vi "子VI-数据库显示.vi"(10 "数据库保存路径":path, 11 "表名":string) -> (2 "Table":string[][](table) caption="表格")   [LabVIEW 2018]
uses:
  <vilib>/addons/database/_DB Variant To Data/Database Variant To Data.xnode
  <vilib>/addons/database/Connection.llb/DB Tools Open Connec (String).vi
  <vilib>/addons/database/NI_Database_API.lvlib
panel:
  out "data":string[][](array[string])
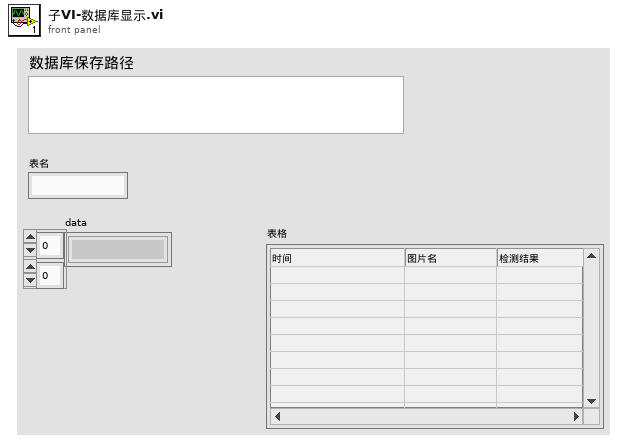
[diagram p1: front panel]
types:
  T1 = typedef "NI_Database_API.lvlib/Conn ObjectReference.ctl" = refnum<k1>
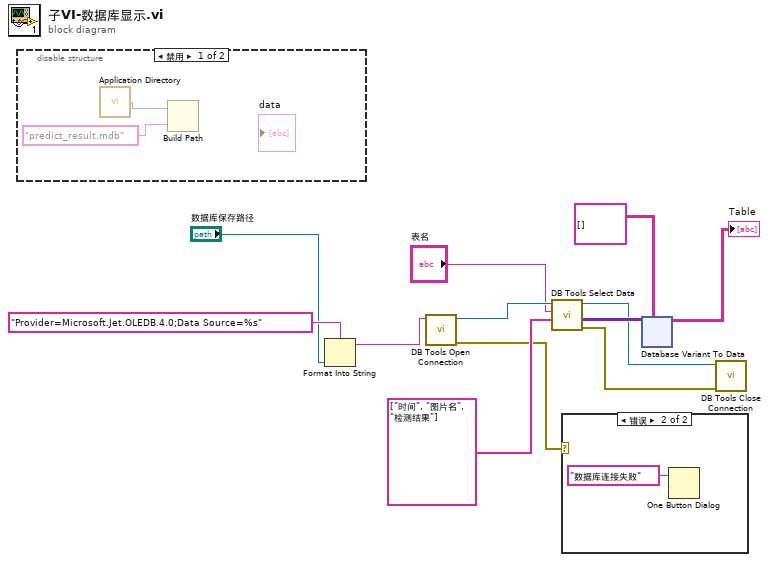
[diagram p0: block diagram]
diagram:
  n1 = disable-structure shown="禁用" {
    frame Disabled {
      n2 = call <vilib>:"Application Directory.vi"() -> ("Application Directory"=w14:path)
      n3 = Build Path(base path=w14, name or relative path="predict_result.mdb" ("名称或相对路径")) -> ()  [unwired: 1 out]
    }
    frame Enabled {
    }
  }
  n4 = Format Into String(format string="Provider=Microsoft.Jet.OLEDB.4.0;Data Source=%s" ("格式字符串"), "数据库保存路径") -> (resulting string=w4:string)  [unwired: 2 in, 1 out]
  n5 = call-poly <vilib>:"DB Tools Open Connection.vi"("connection information"=w4) -> ("error out"=w2:errorcluster, "connection reference"=w12:T1)  [unwired: 7 in]
  n6 = call <vilib>:"DB Tools Select Data.vi"("columns"=string[] ["时间", "图片名", "检测结果"], "table"="表名", "connection reference"=w12) -> ("error out"=w8:errorcluster, "data"=w11:variant[][], "connection reference out"=w9:T1)  [unwired: 3 in]
  n7 = case shown="错误" w2 {
    frame No Error {
    }
    frame Error {
      n8 = One Button Dialog(message="数据库连接失败" ("消息")) -> ()  [unwired: 1 in, 1 out]
    }
  }
  n9 = xnode "Database Variant To Data"("database variant"=w11, "type"=string[][] []) -> ("data"=→"Table":string[][])  [unwired: 1 in, 1 out]
  n10 = call <vilib>:"DB Tools Close Connection.vi"("error in (no error)"=w8, "connection reference"=w9) -> ()  [unwired: 5 in, 1 out]
